vi "SimpleDemoWithEvents.vi"() -> ()   [LabVIEW 2012]
panel:
  out "Data Done":bool
  out "Data Available":bool
  out "NumPoints":i32
  out "Waveform Chart":dbl[](graph)
  out "error out":errorcluster
  in  "SampleRate":sgl=0.1
  in  "Tfinal":sgl=1.0
  in  "Vfinal":sgl=-0.1
  in  "Tinit":sgl=1.0
  in  "Vinit":sgl=0.1
  in  "GAMRYCOMLib.IGamrySignal":refnum<k7>
  in  "GAMRYCOMLib.IGamrySignalStep":refnum<k7>
  in  "GAMRYCOMLib.IGamryDtaqIv":refnum<k7>
  in  "GAMRYCOMLib.IGamryPstat":refnum<k7>
  in  "GAMRYCOMLib.IGamryDeviceList":refnum<k7>
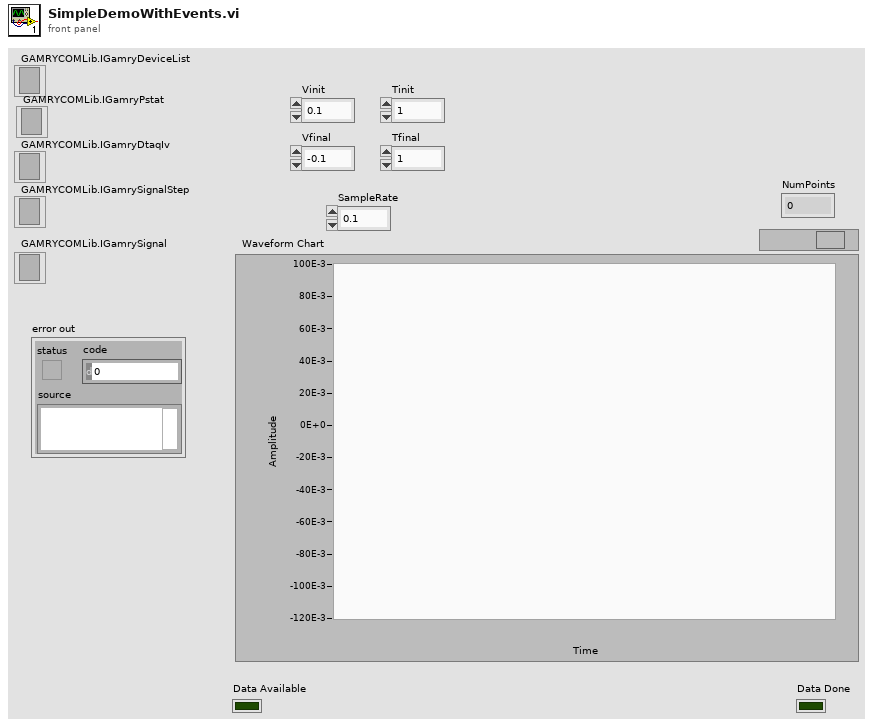
[diagram p1: front panel]
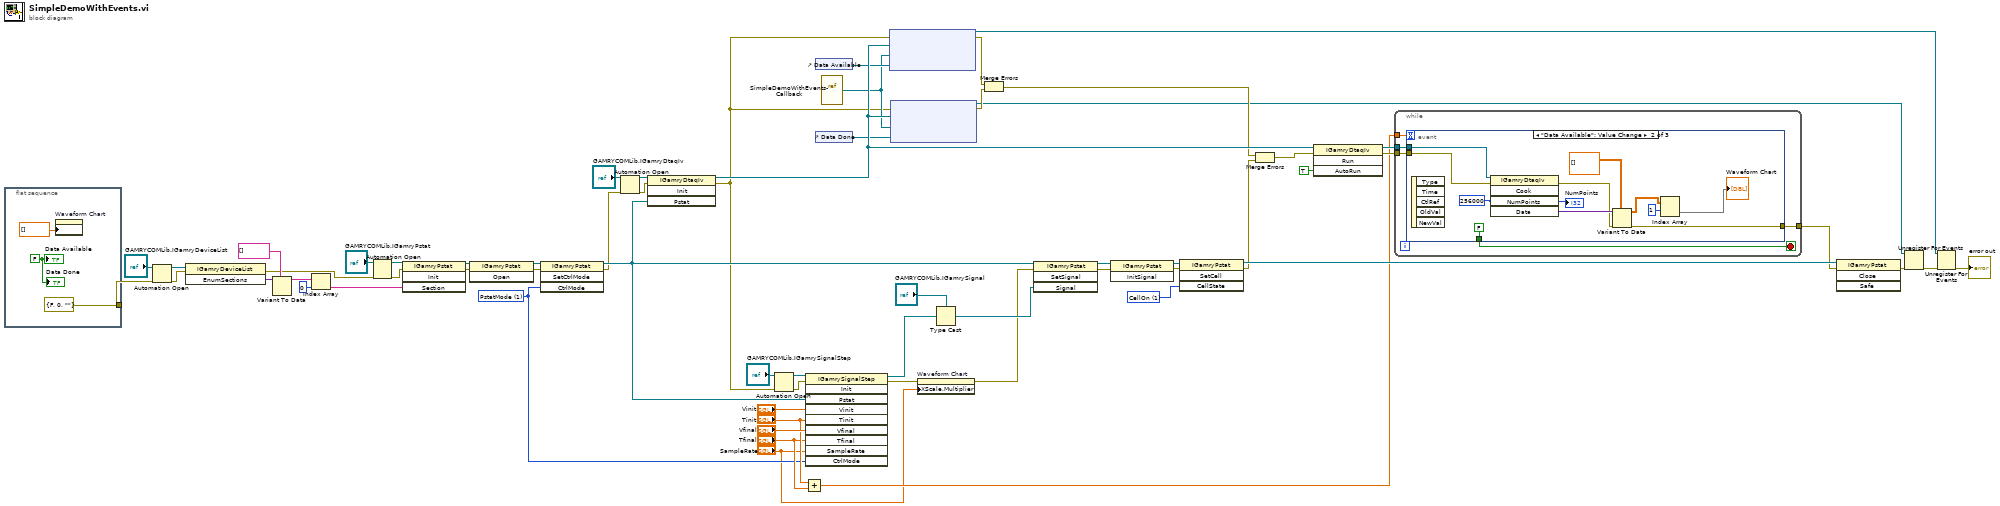
[diagram p0: block diagram]
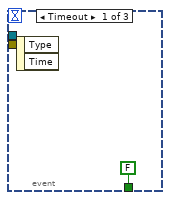
[diagram p2: hidden frame]
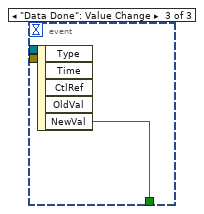
[diagram p3: hidden frame]
diagram:
  w32 = 1 items=["CellOff", "CellOn", "CellMon", "CellRelay"] ("CellState")
  w23 = 1 items=["GstatMode", "PstatMode", "ZRAMode", "FRAMode"] ("CtrlMode")
  n1 = flat-sequence {
    tunnel: [errorcluster {"status"=FALSE, "code"=0, "source"=""} ("error in (no error)")] -> w4
    frame #0 {
      w65 = FALSE ("Data Available")
      n2 = property on="Waveform Chart" class="WFChart (strict)"("History Data"=dbl[] []) -> ()  [unwired: 2 in, 2 out]
      "Data Available" <- w65
      "Data Done" <- w65
    }
  }
  n3 = Automation Open(error in (no error)=w4, Automation Refnum="GAMRYCOMLib.IGamryDeviceList") -> (Automation Refnum=w61:refnum<k7>, error out=w60:errorcluster)  [unwired: 2 in]
  n4 = invoke class="IGamryDeviceList" method="EnumSections"(reference=w61, error in=w60) -> (error out=w46:errorcluster, "EnumSections"=w59:variant)  [unwired: 1 in, 1 out]
  n5 = Variant To Data(type=string[] [], Variant=w59) -> (data=w57:string[])  [unwired: 1 in, 1 out]
  n6 = Index Array(array=w57, index=0) -> (element=w52:string)
  n7 = Automation Open(error in (no error)=w46, Automation Refnum="GAMRYCOMLib.IGamryPstat") -> (Automation Refnum=w54:refnum<k7>, error out=w53:errorcluster)  [unwired: 2 in]
  n8 = invoke class="IGamryPstat" method="Init"(reference=w54, error in=w53, "Section"=w52) -> (reference out=w50:refnum<k7>, error out=w51:errorcluster)  [unwired: 1 in, 2 out]
  n9 = invoke class="IGamryPstat" method="Open"(reference=w50, error in=w51) -> (reference out=w42:refnum<k7>, error out=w41:errorcluster)  [unwired: 1 in, 1 out]
  n10 = invoke class="IGamryPstat" method="SetCtrlMode"(reference=w42, error in=w41, "CtrlMode"=w23) -> (reference out=w40:refnum<k7>, error out=w31:errorcluster)  [unwired: 1 in, 2 out]
  n11 = Automation Open(error in (no error)=w31, Automation Refnum="GAMRYCOMLib.IGamryDtaqIv") -> (Automation Refnum=w48:refnum<k7>, error out=w47:errorcluster)  [unwired: 2 in]
  n12 = invoke class="IGamryDtaqIv" method="Init"(reference=w48, error in=w47, "Pstat"=w40) -> (reference out=w21:refnum<k7>, error out=w15:errorcluster)  [unwired: 1 in, 2 out]
  n13 = Automation Open(error in (no error)=w15, Automation Refnum="GAMRYCOMLib.IGamrySignalStep") -> (Automation Refnum=w44:refnum<k7>, error out=w43:errorcluster)  [unwired: 2 in]
  n14 = Add(x="Tinit", y="Tfinal") -> (x+y=w5:sgl)
  n15 = invoke class="IGamrySignalStep" method="Init"(reference=w44, error in=w43, "Pstat"=w40, "Vinit"="Vinit", "Tinit"="Tinit", "Vfinal"="Vfinal", "Tfinal"="Tfinal", "SampleRate"="SampleRate", "CtrlMode"=w23) -> (reference out=w39:refnum<k7>, error out=w2:errorcluster)  [unwired: 1 in, 8 out]
  n16 = control-ref of="Data Available"() -> (w20:refnum<vi>)
  n17 = control-ref of="Data Done"() -> (w19:refnum<vi>)
  n18 = vi-ref "SimpleDemoWithEvents-Callback.vi"() -> ("vi reference"=w18:refnum<vi>)
  n19 = node(w15, w21, w18, w20) -> (w8:refnum<k27>, w17:errorcluster)  [unwired: 1 in]
  n20 = node(w15, w21, w18, w19) -> (w7:refnum<k27>, w16:errorcluster)  [unwired: 1 in]
  n21 = property on="Waveform Chart" class="WFChart (strict)"(error in=w2, "XScale.Multiplier"="SampleRate") -> (error out=w1:errorcluster)  [unwired: 1 in, 1 out]
  n22 = Type Cast(type="GAMRYCOMLib.IGamrySignal", x=w39) -> (*(type *) &x=w37:refnum<k7>)
  n23 = Merge Errors(w17, w16) -> (w14:errorcluster)
  n24 = invoke class="IGamryPstat" method="SetSignal"(reference=w40, error in=w1, "Signal"=w37) -> (reference out=w36:refnum<k7>, error out=w35:errorcluster)  [unwired: 1 in, 2 out]
  n25 = invoke class="IGamryPstat" method="InitSignal"(reference=w36, error in=w35) -> (reference out=w34:refnum<k7>, error out=w33:errorcluster)  [unwired: 1 in, 1 out]
  n26 = invoke class="IGamryPstat" method="SetCell"(reference=w34, error in=w33, "CellState"=w32) -> (reference out=w25:refnum<k7>, error out=w13:errorcluster)  [unwired: 1 in, 2 out]
  n27 = Merge Errors(w14, w13) -> (w12:errorcluster)
  n28 = invoke class="IGamryDtaqIv" method="Run"(reference=w21, error in=w12, "AutoRun"=TRUE) -> (reference out=w26:refnum<k7>, error out=w6:errorcluster)  [unwired: 1 in, 2 out]
  n29 = while {
    tunnel: w26 -> [w70]
    tunnel: [w69] -> w24
    tunnel: w6 -> [w68]
    tunnel: w5 -> [w66]
    stop <- w67 stop-if-true
    n30 = event shown="[1] \"Data Available\": Value Change" {
      selector: _ -> [_ _ _]
      dyn-events: _ -> [_ _ _]
      timeout: w66 -> [_ _ _]
      tunnel: w68 -> [_ w83 _]
      tunnel: w70 -> [_ w82 _]
      tunnel: [_ w78 _] -> w69
      tunnel: [FALSE ("NewVal") FALSE ("NewVal") w84] -> w67
      event Timeout {
        n31 = event-data() -> ()  [unwired: 1 in, 2 out]
      }
      event "Data Available": Value Change {
        n32 = event-data() -> ()  [unwired: 1 in, 5 out]
        n33 = invoke class="IGamryDtaqIv" method="Cook"(reference=w82, error in=w83, "NumPoints"=256000) -> (error out=w79:errorcluster, "NumPoints"=→"NumPoints":i32, "Data"=w80:variant)  [unwired: 2 in, 2 out]
        n34 = Variant To Data(error in=w79, type=dbl[][] [], Variant=w80) -> (data=w75:dbl[][], error out=w78:errorcluster)
        n35 = Index Array(array=w75, index (row)=1) -> (element=→"Waveform Chart":dbl[])  [unwired: 1 in]
      }
      event "Data Done": Value Change {
        n36 = event-data() -> ("NewVal"=w84:bool)  [unwired: 1 in, 4 out]
      }
    }
  }
  n37 = invoke class="IGamryPstat" method="Close"(reference=w25, error in=w24) -> (error out=w10:errorcluster)  [unwired: 2 in, 3 out]
  n38 = Unregister For Events(event registration refnum=w7, error in=w10) -> (error out=w11:errorcluster)
  n39 = Unregister For Events(event registration refnum=w8, error in=w11) -> (error out=→"error out":errorcluster)
